vi "Get Type.vi"(8 "error in (no error)":errorcluster, 11 "Circuit Board in":refnum<class "Circuit Board.lvclass">) -> (0 "error out":errorcluster, 2 "Item Type":T1, 3 "Circuit Board out":refnum<class "Circuit Board.lvclass">)   [LabVIEW 2020, in "Circuit Board.lvclass"]
uses:
  Circuit Board.lvclass
  Item/Item Type.ctl
  Item/Item.lvclass
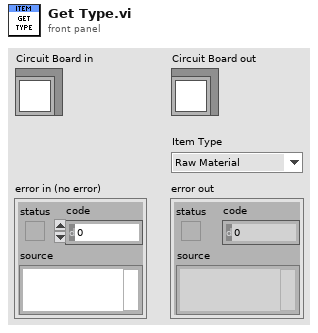
[diagram p1: front panel]
types:
  T1 = typedef "Item.lvclass/Item Type.ctl" = enum16{"Raw Material", "Component", "Module", "Product"}
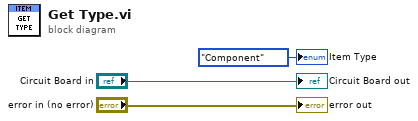
[diagram p0: block diagram]
diagram:
  "error out" <- "error in (no error)"
  "Circuit Board out" <- "Circuit Board in"
  "Item Type" <- Item_Type."Component" ("Item Type")
